vi "MCP3422 Config.vi"(0 "VISA Refnum in":refnum<visa-resource-name>, 5 "Channel selection":u8, 7 "Gain selection":u8, 9 "Sample rate selection":u8, 11 "error in (no error)":errorcluster, 12 "Continuous conversion":u8, 13 "Initiate conversion":u8) -> (4 "VISA Refnum out":refnum<visa-resource-name>, 15 "error out":errorcluster)   [LabVIEW 2015]
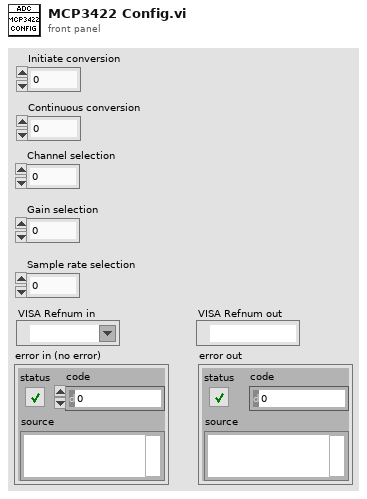
[diagram p1: front panel]
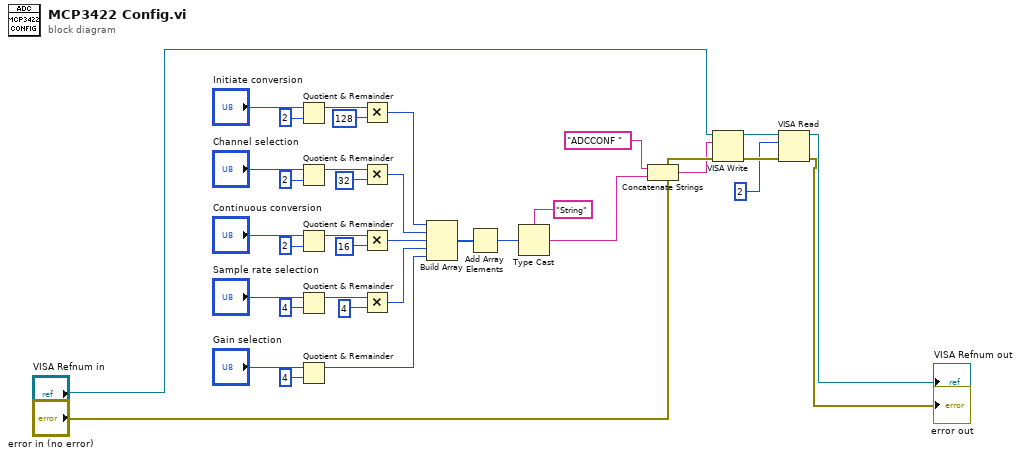
[diagram p0: block diagram]
diagram:
  n1 = Quotient & Remainder(x="Initiate conversion", y=u8 2) -> (x-y*floor(x/y)=w11:u8)  [unwired: 1 out]
  n2 = Quotient & Remainder(x="Channel selection", y=u8 2) -> (x-y*floor(x/y)=w18:u8)  [unwired: 1 out]
  n3 = Quotient & Remainder(x="Continuous conversion", y=u8 2) -> (x-y*floor(x/y)=w15:u8)  [unwired: 1 out]
  n4 = Quotient & Remainder(x="Sample rate selection", y=u8 4) -> (x-y*floor(x/y)=w22:u8)  [unwired: 1 out]
  n5 = Quotient & Remainder(x="Gain selection", y=u8 4) -> (x-y*floor(x/y)=w8:u8)  [unwired: 1 out]
  n6 = Multiply(x=w11, y=u8 128) -> (x*y=w4:u8)
  n7 = Multiply(x=w18, y=u8 32) -> (x*y=w5:u8)
  n8 = Multiply(x=w15, y=u8 16) -> (x*y=w6:u8)
  n9 = Multiply(x=w22, y=u8 4) -> (x*y=w7:u8)
  n10 = Build Array(w4, w5, w6, w7, w8) -> (w3:u8[])
  n11 = Add Array Elements(numeric array=w3) -> (sum=w2:u8)
  n12 = Type Cast(type="String", x=w2) -> (*(type *) &x=w1:string)
  n13 = Concatenate Strings("ADCCONF " ("string"), w1) -> (w33:string)
  n14 = VISA Write(VISA resource name="VISA Refnum in", write buffer=w33, error in (no error)="error in (no error)") -> (VISA resource name out=w32:refnum<visa-resource-name>, error out=w31:errorcluster)  [unwired: 1 out]
  n15 = VISA Read(VISA resource name=w32, byte count=u32 2, error in (no error)=w31) -> (VISA resource name out=→"VISA Refnum out":refnum<visa-resource-name>, error out=→"error out":errorcluster)  [unwired: 2 out]
